vi "createCursors.vi"(4 "xAxisFormat":u16, 5 "plotNumber":i32, 7 "howManyPoints":u32=10, 8 "step, ms":dbl=1.0, 9 "sourceGraph":refnum<vi>, 10 "write":bool, 11 "dataCutCluster":refnum<vi>) -> (2 "listOfProfilesPath":path[](array[path]))   [LabVIEW 2014]
uses:
  <vilib>/Waveform/WDTOps.llb/WDT Get XY Value DBL.vi
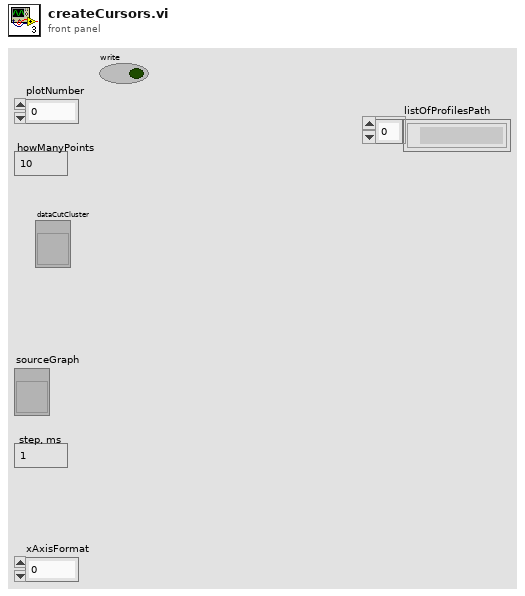
[diagram p1: front panel]
types:
  T1 = cluster{"Name":string, "Color":u32, "Style":u8, "Point Style":u8, "Name Visible":bool, "Allow Drag":bool, "Cursor Mode":u32, "Plot":i32, "Index":i32, "Position":cluster{"X":dbl, "Y":dbl}, "X Scale":u32, "Y Scale":u32, "Watch Plots":i32[], "Watch All Plots":bool, "Plot Area":i32, "Label Offset":cluster{"X":dbl, "Y":dbl}}
  T2 = typedef "LVCursorListTypeDef.ctl" = cluster{"Name":string, "Color":u32, "Style":u8, "Point Style":u8, "Name Visible":bool, "Allow Drag":bool, "Cursor Mode":u32, "Plot":i32, "Index":i32, "Position":cluster{"X":dbl, "Y":dbl}, "X Scale":u32, "Y Scale":u32, "Watch Plots":i32[], "Watch All Plots":bool, "Plot Area":i32, "Label Offset":cluster{"X":dbl, "Y":dbl}}[]
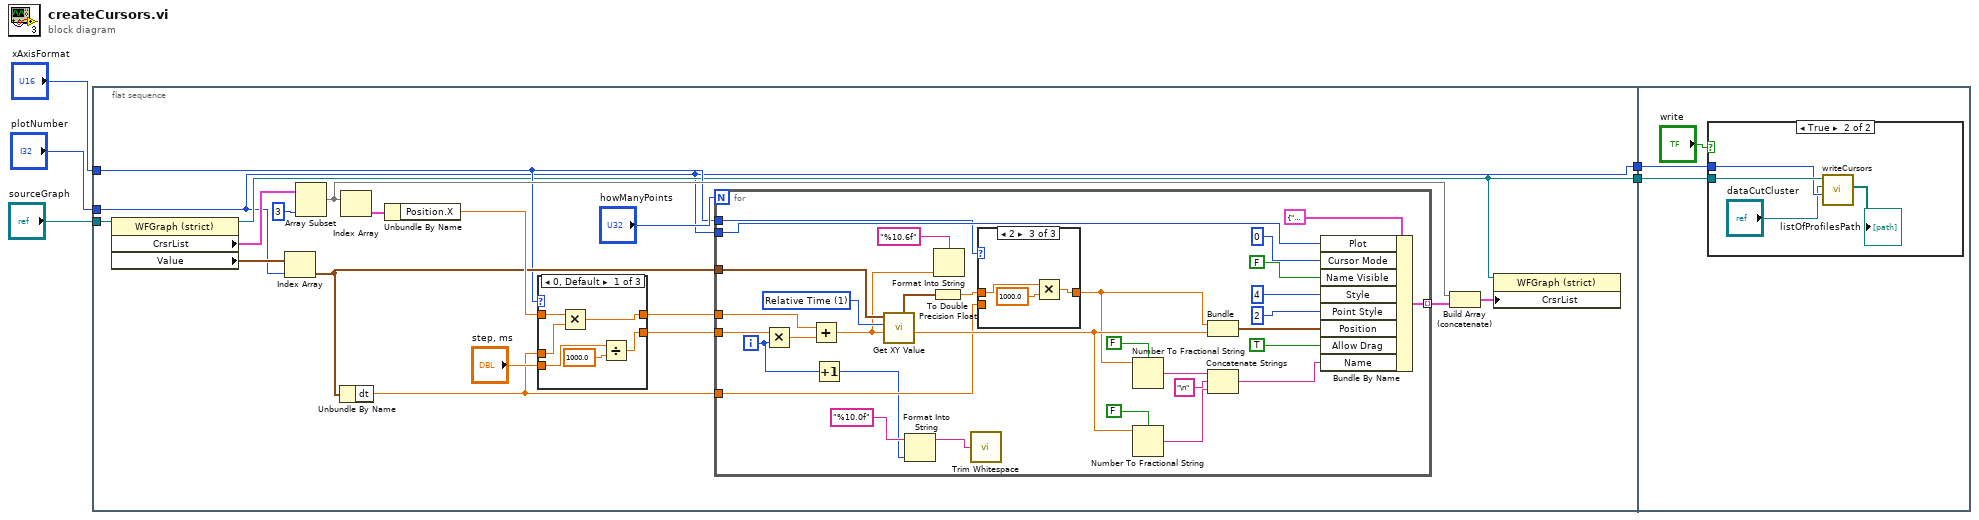
[diagram p0: block diagram]
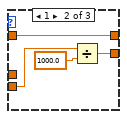
[diagram p2: hidden frame]
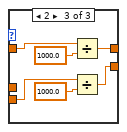
[diagram p3: hidden frame]
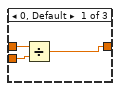
[diagram p4: hidden frame]
diagram:
  n1 = flat-sequence {
    tunnel: "sourceGraph" -> [w21]
    tunnel: "plotNumber" -> [w6]
    tunnel: "xAxisFormat" -> [w8]
    tunnel: [w7] -> w2
    tunnel: [w6] -> w1
    tunnel: w2 -> [w81]
    tunnel: w1 -> [w80]
    frame #0 {
      n2 = property on="Property Node" class="WFGraph (strict)"(reference=w21) -> (reference out=w7:refnum<vi>, "CrsrList"=w23:T2, "Value"=w15:waveform(dbl)[])  [unwired: 1 in, 1 out]
      n3 = Index Array(array=w15, index=w6) -> (element=w13:waveform(dbl))
      n4 = Array Subset(array=w23, length=3) -> (w19:T2)  [unwired: 1 in]
      n5 = Unbundle By Name(w13) -> ("dt"=w9:dbl)
      n6 = Index Array(array=w19) -> (element=w20:T1)  [unwired: 1 in]
      n7 = Unbundle By Name(w20) -> ("Position.X"=w14:dbl)
      n8 = case shown="0, Default" w8 {
        tunnel: w14 -> [w29 w33 w39]
        tunnel: "step, ms" -> [w25 w31 w35]
        tunnel: w9 -> [w28 _ _]
        tunnel: [w27 w33 w37] -> w12
        tunnel: [w24 w30 w34] -> w11
        frame 0, Default {
          n9 = Multiply(x=w29, y=w28) -> (x*y=w27:dbl)
          n10 = Divide(x=w25, y=1000.0) -> (x/y=w24:dbl)
        }
        frame 1 {
          n11 = Divide(x=w31, y=1000.0) -> (x/y=w30:dbl)
        }
        frame 2 {
          n12 = Divide(x=w39, y=1000.0) -> (x/y=w37:dbl)
          n13 = Divide(x=w35, y=1000.0) -> (x/y=w34:dbl)
        }
      }
      n14 = for {
        N: "howManyPoints" -> [_]
        tunnel: w12 -> [w66]
        tunnel: [w65] -> w18 mode=indexing
        tunnel: w11 -> [w64]
        tunnel: w13 -> [w61]
        tunnel: w6 -> [w56]
        tunnel: w8 -> [w49]
        tunnel: w9 -> [w46]
        i -> [w44]
        w57 = u16 1 items=["Samples", "Relative Time"] ("Y position format")
        n15 = Multiply(x=w64, y=w44) -> (x*y=w60:dbl)
        n16 = Add(x=w66, y=w60) -> (x+y=w45:dbl)
        n17 = Increment(x=w44) -> (x+1=w42:i32)
        n18 = call-poly <vilib>:"Get XY Value.vi"("Y position"=w45, "Y position format"=w57, "waveform in"=w61) -> ("Y value"=w50:dbl, "X value"=w58:timestamp)  [unwired: 4 in, 3 out]
        n19 = Format Into String(format string="%10.0f", w42) -> (resulting string=w41:string)  [unwired: 2 in, 1 out]
        n20 = To Double Precision Float(number=w58) -> (double precision float=w48:dbl)
        n21 = Format Into String(format string="%10.6f", w45) -> ()  [unwired: 2 in, 2 out]
        n22 = call <vilib>:"Trim Whitespace.vi"("string"=w41) -> ()  [unwired: 1 in, 1 out]
        n23 = case shown="2" w49 {
          tunnel: w48 -> [w74 w75 w78]
          tunnel: [w72 w75 w76] -> w47
          tunnel: w46 -> [w73 _ _]
          frame 0, Default {
            n24 = Divide(x=w74, y=w73) -> (x/y=w72:dbl)
          }
          frame 1 {
          }
          frame 2 {
            n25 = Multiply(x=w78, y=1000.0) -> (x*y=w76:dbl)
          }
        }
        n26 = Number To Fractional String(use system decimal point (T)=FALSE, number=w47) -> (F-format string=w54:string)  [unwired: 2 in]
        n27 = Number To Fractional String(use system decimal point (T)=FALSE, number=w50) -> (F-format string=w51:string)  [unwired: 2 in]
        n28 = Bundle(w47, "Y value"=w50) -> (w59:cluster{dbl, "Y value":dbl})  [unwired: 1 in]
        n29 = Concatenate Strings(w54, "\n" ("string"), w51) -> (w40:string)
        n30 = Bundle By Name(cluster=T1 {"Name"="", "Color"=0, "Style"=0, "Point Style"=0, "Name Visible"=FALSE, "Allow Drag"=FALSE, "Cursor Mode"=0, "Plot"=0, "Index"=0, "Position"={"X"=0.0, "Y"=0.0}, "X Scale"=0, "Y Scale"=0, "Watch Plots"=[], "Watch All Plots"=FALSE, "Plot Area"=0, "Label Offset"={"X"=0.0, "Y"=0.0}} ("element"), "Plot"=w56, "Cursor Mode"=u32 0, "Name Visible"=FALSE ("Watch All Plots"), "Style"=u8 4, "Point Style"=u8 2, "Position"=w59, "Allow Drag"=TRUE, "Name"=w40) -> (w65:T1)
      }
      n31 = Build Array (concatenate)(w19, w18) -> (w17:T2)
      n32 = property on="Property Node" class="WFGraph (strict)"(reference=w7, "CrsrList"=w17) -> ()  [unwired: 1 in, 2 out]
    }
    frame #1 {
      n33 = case shown="True" "write" {
        tunnel: w81 -> [_ w85]
        tunnel: w80 -> [_ w84]
        frame False {
        }
        frame True {
          n34 = call "writeCursors.vi"("plotNumber"=w84, "dataCutCluster"="dataCutCluster", "WaveformGraph in"=w85) -> ("listOfProfiles"=→"listOfProfilesPath":path[])  [unwired: 7 in, 1 out]
        }
      }
    }
  }
